vi "create arm trigger channel.vi"(8 "error in":errorcluster, 11 "TDMS datalogger configuration":refnum<class "TDMS datalogger configuration.lvclass">) -> (0 "error out":errorcluster, 2 "arm trigger channel name":string, 3 "enable channel":refnum<class "TBM channel.lvclass">)   [LabVIEW 2015, in "TDMS datalogger configuration.lvclass"]
uses:
  TDMS datalogger configuration.lvclass
  <vilib>/NI/Tag Bus Module Framework/channel/TBM channel.lvclass
  <vilib>/NI/Tag Bus/tag/Data Type.ctl
  <vilib>/NI/Tag Bus Module Framework/channel/channel classification.ctl
  <vilib>/NI/Configuration Framework/serializable configuration/NISE_CEF_serializable configuration.lvclass/NISE_CEF_serializable configuration.ctl
  <vilib>/Utility/LVClass/Get LV Class Name.vi
  <vilib>/NI/Configuration Framework/error generator/NISE_error generator.vi
  <vilib>/NI/Tag Bus/tag/default value polymorphs/write default value Boolean.vi
  <vilib>/NI/Tag Bus/tag/tag descriptor.lvclass
  <vilib>/NI/Configuration Framework/serializable configuration/NISE_CEF_serializable configuration.lvclass
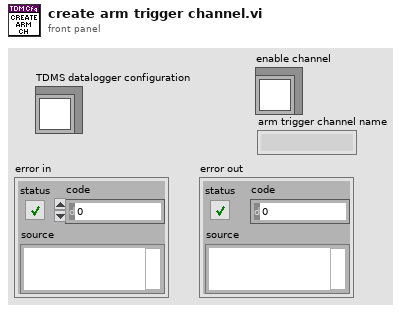
[diagram p1: front panel]
types:
  T1 = typedef "TBM channel.lvclass/channel classification.ctl" = enum16{"input data", "output data", "processing parameter", "processing result"}
  T2 = typedef "tag bus.lvlib/tag descriptor.lvclass/Data Type.ctl" = enum16{"Double", "Single", "I64", "I32", "I16", "I8", "U64", "U32", "U16", "U8", "Boolean", "String", "Array of Double", "Array of Single", "Array of I64", "Array of I32", "Array of I16", "Array of I8", "Array of U64", "Array of U32", "Array of U16", "Array of U8", "Array of Boolean", "Array of String"}
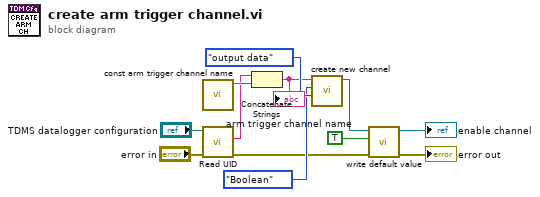
[diagram p0: block diagram]
diagram:
  n1 = call "const arm trigger channel name.vi"() -> ("arm trigger channel"=w12:string)  [unwired: 11 in]
  n2 = call <vilib>:"Read UID.vi"("error in"="error in", "configuration in"="TDMS datalogger configuration") -> ("error out"=w4:errorcluster, "instance id"=w1:string)  [unwired: 7 in, 1 out]
  n3 = Concatenate Strings(w1, w12) -> (w2:string)
  "arm trigger channel name" <- w2
  n4 = call <vilib>:"create new channel.vi"("channel classification"=channel_classification."output data", "data type"=Data_Type."Boolean", "channel name"=w2) -> ("channel"=w8:refnum<class "TBM channel.lvclass">)  [unwired: 8 in]
  n5 = call-poly <vilib>:"write default value.vi"("error in"=w4, "default value"=TRUE, "system tag in"=w8) -> ("error out"=→"error out":errorcluster, "system tag out"=→"enable channel":refnum<class "TBM channel.lvclass">)  [unwired: 7 in]
